vi "Initialize.vi"(8 "error in (no error)":errorcluster, 10 "Subpanel.lvclass":refnum<class "Subpanel.lvclass">, 11 "Sub Panel":refnum<vi>) -> (0 "error out":errorcluster, 3 "Subpanel out":refnum<class "Subpanel.lvclass">)   [LabVIEW 2019, in "Subpanel.lvclass"]
uses:
  Subpanel.lvclass
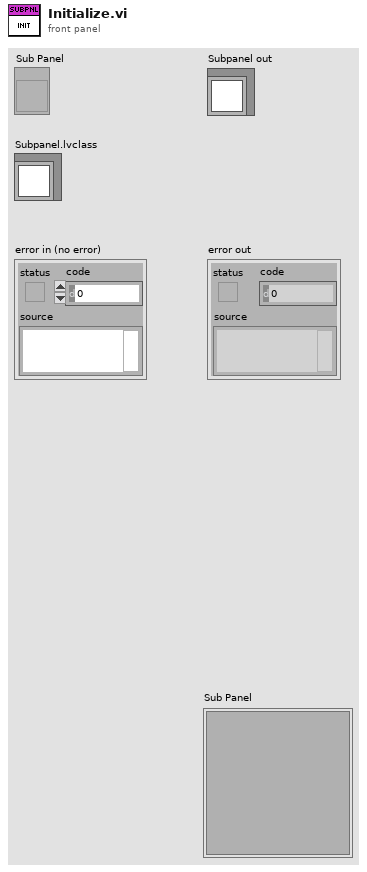
[diagram p1: front panel]
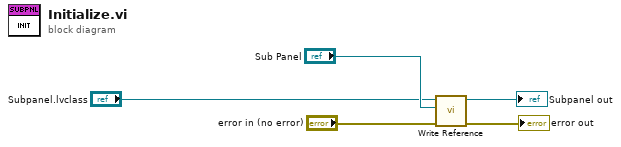
[diagram p0: block diagram]
diagram:
  n1 = call-dynamic "Write Reference.vi"("error in (no error)"="error in (no error)", "Reference"="Sub Panel", "Subpanel in"="Subpanel.lvclass") -> ("error out"=→"error out":errorcluster, "Subpanel out"=→"Subpanel out":refnum<class "Subpanel.lvclass">)  [unwired: 7 in]
